vi "nirviMacc.vi"(1 "sum":i32, 2 "y":i16, 3 "x":i16) -> (0 "x*y+sum":i32)   [LabVIEW 2017]
doc: "Multiplies two 16-bit numbers and adds the result to the sum input to yield the 32-bit x*y+sum value. This operation is carried out using saturation arithmetic to avoid integer overflow by returning a maximum or minimum value."
uses:
  <vilib>/rvi/Arithmetic/AddSubMult/XNode/nirviSatArithmetic.xnode
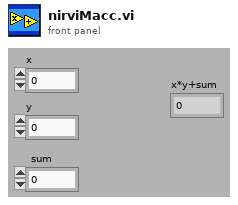
[diagram p1: front panel]
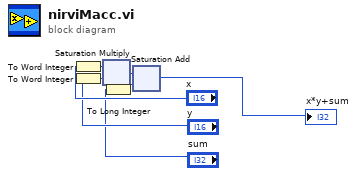
[diagram p0: block diagram]
diagram:
  n1 = To Word Integer(number="x") -> (16bit integer=w1:i16)
  n2 = To Word Integer(number="y") -> (16bit integer=w2:i16)
  n3 = xnode "Saturation Multiply"("x"=w1, "y"=w2) -> ("x*y"=w6:i32)
  n4 = To Long Integer(number="sum") -> (32bit integer=w3:i32)
  n5 = xnode "Saturation Add"("x"=w6, "y"=w3) -> ("x+y"=→"x*y+sum":i32)
